vi "activeXtest.vi"() -> ()   [LabVIEW 2016]
panel:
  out "error out":errorcluster
  in  "Excel._Application":refnum<k7>
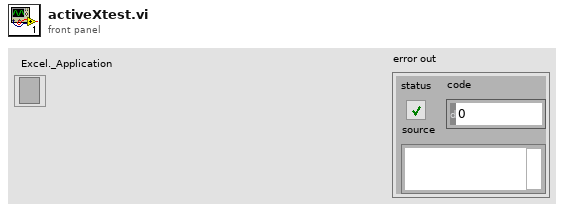
[diagram p1: front panel]
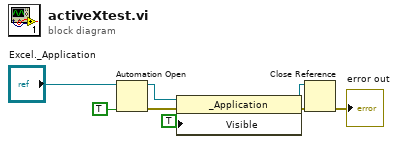
[diagram p0: block diagram]
diagram:
  n1 = Automation Open(Automation Refnum="Excel._Application", 9:TRUE ("open new instance (false)")) -> (Automation Refnum=w6:refnum<k7>, error out=w7:errorcluster)  [unwired: 2 in]
  n2 = property class="_Application"(reference=w6, error in=w7, "Visible"=TRUE) -> (reference out=w5:refnum<k7>, error out=w4:errorcluster)
  n3 = Close Reference(reference=w5, error in (no error)=w4) -> (error out=→"error out":errorcluster)
